vi "BS tug to string.vi"(1 "Tug location array":T1(array[cluster])) -> (0 "tug location string":string)   [LabVIEW 2012]
doc: "This VI receives the tug location as an array of clusters and creates a single string with the data."
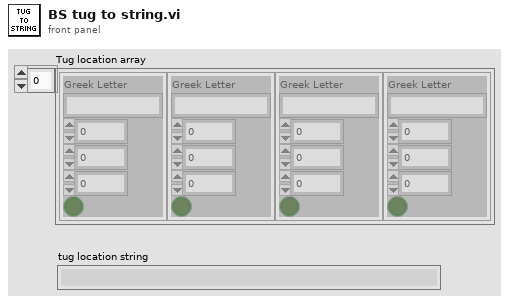
[diagram p1: front panel]
types:
  T1 = cluster{"Greek Letter":string, i16, i16, i16, bool}[]
  T2 = cluster{"Greek Letter":string, i16, i16, i16, bool}
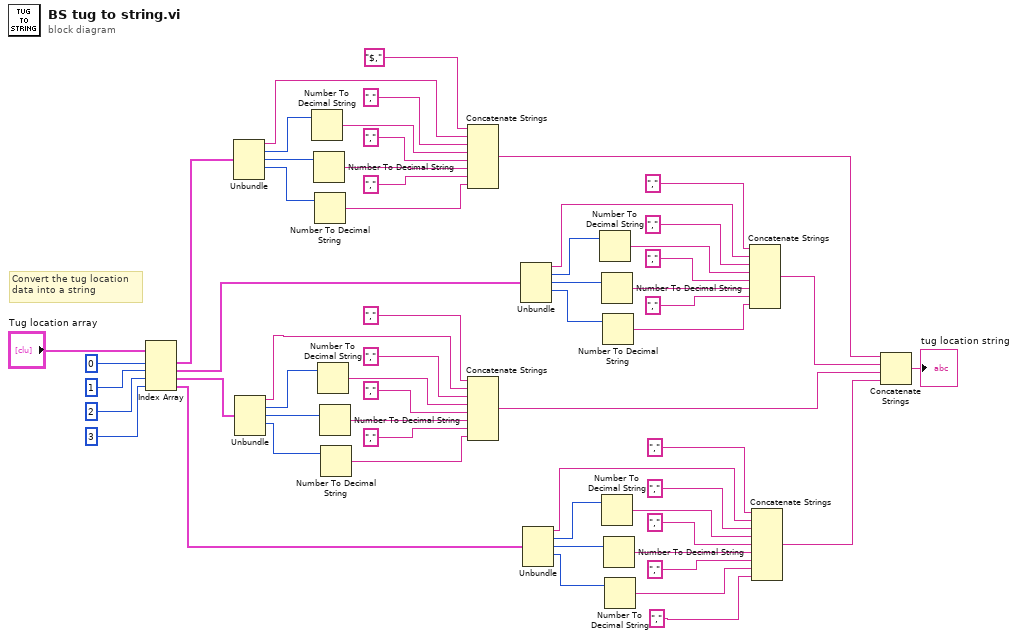
[diagram p0: block diagram]
diagram:
  # "Convert the tug location\ndata into a string"
  n1 = Index Array(array="Tug location array", index #1=0 ("index"), index #2=1 ("index"), index #3=2 ("index"), index #4=3 ("index")) -> (element #1=w54:T2, element #2=w53:T2, element #3=w52:T2, element #4=w51:T2)
  n2 = Unbundle(w54) -> ("Greek Letter"=w32:string, w50:i16, w49:i16, w48:i16)  [unwired: 1 out]
  n3 = Unbundle(w52) -> ("Greek Letter"=w16:string, w15:i16, w14:i16, w13:i16)  [unwired: 1 out]
  n4 = Number To Decimal String(number=w50) -> (decimal integer string=w47:string)  [unwired: 1 in]
  n5 = Number To Decimal String(number=w49) -> (decimal integer string=w45:string)  [unwired: 1 in]
  n6 = Number To Decimal String(number=w48) -> (decimal integer string=w43:string)  [unwired: 1 in]
  n7 = Number To Decimal String(number=w15) -> (decimal integer string=w27:string)  [unwired: 1 in]
  n8 = Number To Decimal String(number=w14) -> (decimal integer string=w25:string)  [unwired: 1 in]
  n9 = Number To Decimal String(number=w13) -> (decimal integer string=w23:string)  [unwired: 1 in]
  n10 = Concatenate Strings("$,", w32, ",", w47, ",", w45, ",", w43) -> (w5:string)
  n11 = Concatenate Strings(",", w16, ",", w27, ",", w25, ",", w23) -> (w3:string)
  n12 = Unbundle(w53) -> ("Greek Letter"=w30:string, w35:i16, w36:i16, w34:i16)  [unwired: 1 out]
  n13 = Unbundle(w51) -> ("Greek Letter"=w11:string, w10:i16, w9:i16, w8:i16)  [unwired: 1 out]
  n14 = Number To Decimal String(number=w35) -> (decimal integer string=w41:string)  [unwired: 1 in]
  n15 = Number To Decimal String(number=w36) -> (decimal integer string=w39:string)  [unwired: 1 in]
  n16 = Number To Decimal String(number=w10) -> (decimal integer string=w21:string)  [unwired: 1 in]
  n17 = Number To Decimal String(number=w34) -> (decimal integer string=w37:string)  [unwired: 1 in]
  n18 = Number To Decimal String(number=w9) -> (decimal integer string=w19:string)  [unwired: 1 in]
  n19 = Number To Decimal String(number=w8) -> (decimal integer string=w17:string)  [unwired: 1 in]
  n20 = Concatenate Strings(",", w30, ",", w41, ",", w39, ",", w37) -> (w4:string)
  n21 = Concatenate Strings(",", w11, ",", w21, ",", w19, ",", w17, ",") -> (w2:string)
  n22 = Concatenate Strings(w5, w4, w3, w2) -> (→"tug location string":string)
